vi "Enqueue.vi"(8 "error in (no error)":errorcluster, 10 "Data":variant, 11 "State":T1) -> (0 "error out":errorcluster)   [LabVIEW 2018, in "template.lvlib"]
uses:
  template.lvlib
  ctl/Module - State.ctl
  ctl/Module Queue - Action.ctl
  ctl/Module - Message.ctl
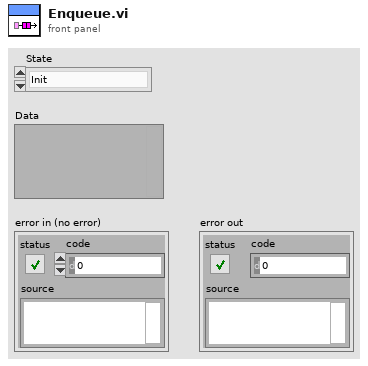
[diagram p1: front panel]
types:
  T1 = typedef "template.lvlib/Module - State.ctl" = enum16{"Init", "Idle", "Error", "Close"}
  T2 = typedef "template.lvlib/Module - Message.ctl" = cluster{"State":T1, "Data":variant}
  T3 = typedef "template.lvlib/Module Queue - Action.ctl" = enum16{"Create", "Get", "Destroy"}
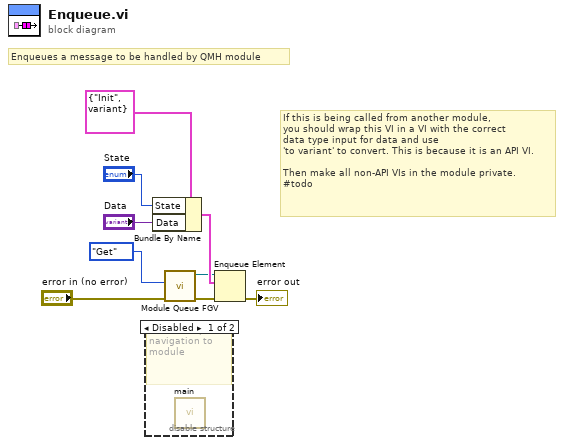
[diagram p0: block diagram]
diagram:
  # "If this is being called from another module,\nyou should wrap this VI in a VI with the correct\ndata type input for data and use\n'to variant' to convert. This is because it is an API VI.\n\nThen make all non-API VIs in the module private.\n#todo"
  # "Enqueues a message to be handled by QMH module"
  n1 = disable-structure shown="Disabled" {
    frame Disabled {
      # "For developer:\nnavigation to module"
      n2 = call "main.vi"() -> ()  [unwired: 11 in, 1 out]
    }
    frame Enabled {
    }
  }
  n3 = Bundle By Name(cluster=T2 {"State"=enum."Init", "Data"=variant} ("element"), "State"="State", "Data"="Data") -> (w4:T2)
  n4 = call "Module Queue FGV.vi"("Error in"="error in (no error)", "Action"=Module_Queue_-_Action."Get") -> ("Error out"=w3:errorcluster, "Queue ref"=w2:refnum<queue>)  [unwired: 8 in]
  n5 = Enqueue Element(queue=w2, element=w4, error in (no error)=w3) -> (error out=→"error out":errorcluster)  [unwired: 1 in, 2 out]
